vi "status of pump.vi"() -> ()   [LabVIEW 2020]
panel:
  in  "status of pump":bool
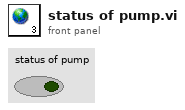
[diagram p1: front panel]
diagram:
